vi "SetParam.vi"(8 "error in (no error)":errorcluster caption="entrée d'erreur (pas d'erreur)", 10 "TestTrain":T1={"test_size"=-1.0, "train_size"=-1.0, "random_state"=-1, "shuffle"=TRUE, "stratify"=[]} {"random_state" min=-1; "train_size" min=-1.0; "test_size" min=-1.0}, 11 "TrainTest.lvclass":refnum<class "TrainTest.lvclass">) -> (0 "error out":errorcluster caption="sortie d'erreur", 3 "TrainTest.lvclass":refnum<class "TrainTest.lvclass">)   [LabVIEW 2020, in "TrainTest.lvclass"]
doc: "Set Parameters"
uses:
  TrainTest.lvclass
  TrainTest.lvclass/TrainTest.ctl
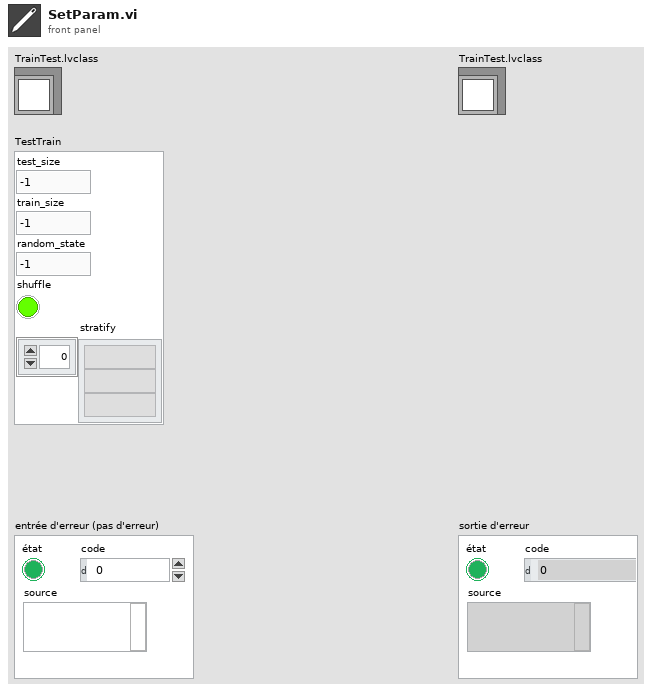
[diagram p1: front panel]
types:
  T1 = cluster{"test_size":dbl, "train_size":dbl, "random_state":i32, "shuffle":bool, "stratify":string[]}
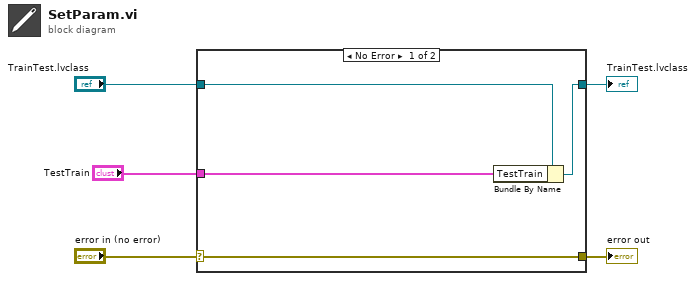
[diagram p0: block diagram]
diagram:
  n1 = case shown="No Error" "error in (no error)" {
    selector: "error in (no error)" -> [w9 w10]
    tunnel: [w9 w10] -> w4
    tunnel: [w7 w11] -> w2
    tunnel: "TrainTest.lvclass" -> [w8 w11]
    tunnel: "TestTrain" -> [w6 _]
    frame No Error {
      n2 = Bundle By Name(cluster=w8, "TestTrain"=w6) -> (w7:refnum<class "TrainTest.lvclass">)
    }
    frame Error {
    }
  }
  "error out" <- w4
  "TrainTest.lvclass" <- w2
